vi "Duplicate Control Names--error.vi"(11 "Control Name":string) -> (0 "error out":errorcluster)   [LabVIEW 2020, in "MacroAssert.lvlib"]
uses:
  MacroAssert.lvlib
  <vilib>/ErrorRing/Error Ring.xnode
  <vilib>/Utility/error.llb/Error Cluster From Error Code.vi
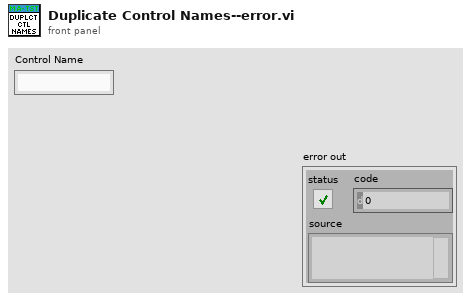
[diagram p1: front panel]
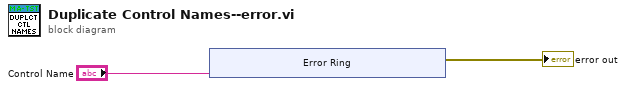
[diagram p0: block diagram]
diagram:
  n1 = xnode "Error Ring"("parameter 0"="Control Name") -> ("error out"=→"error out":errorcluster)
